vi "User_Change_Password.vi"(11 "User_Name":string caption="用  户  名") -> ()   [LabVIEW 2020]
panel:
  in  "Confirm Password":string caption="确认密码"
  in  "New Password":string caption="新  密  码"
  in  "Last Password":string caption="旧  密  码"
  in  "Ok":bool
  # "修改密码"
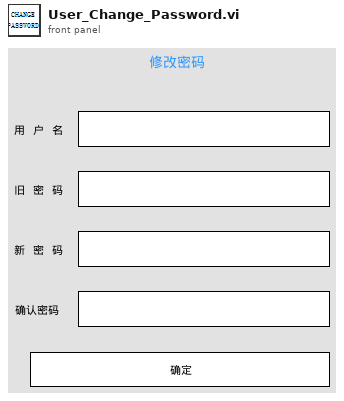
[diagram p1: front panel]
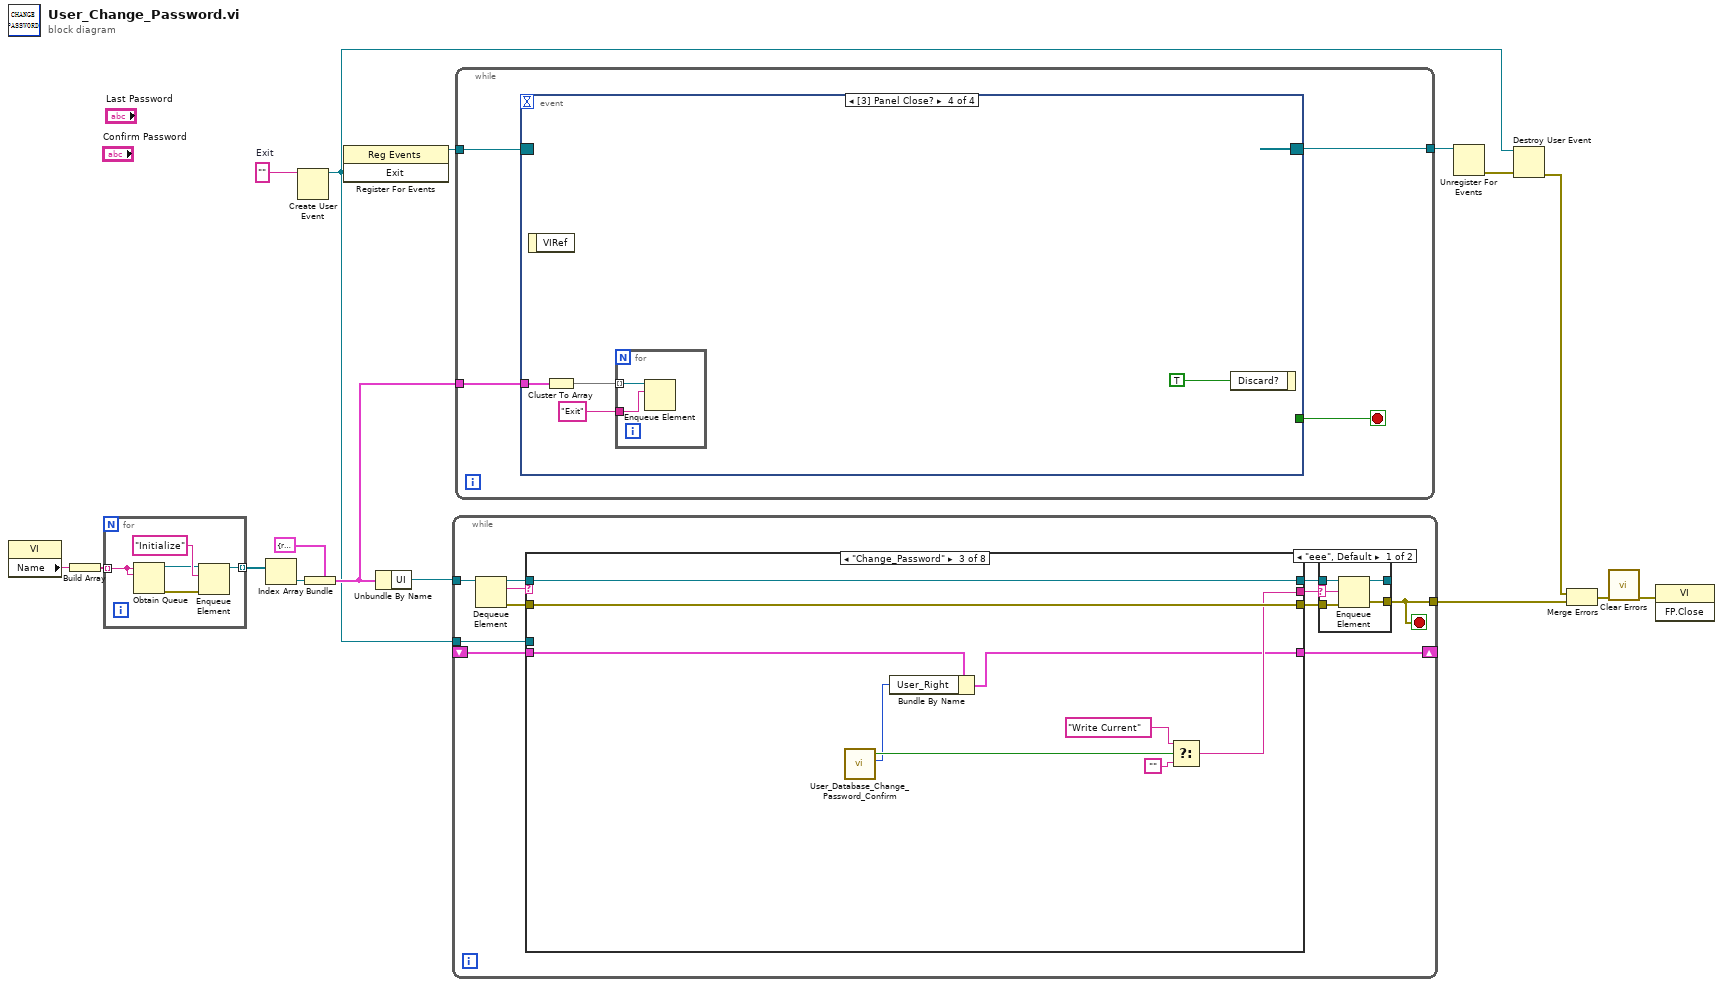
[diagram p0: block diagram]
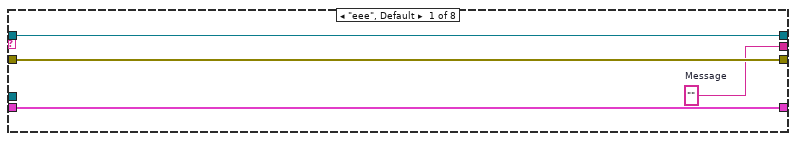
[diagram p3: hidden frame]
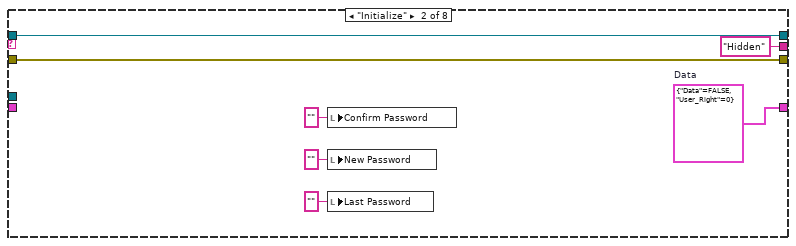
[diagram p4: hidden frame]
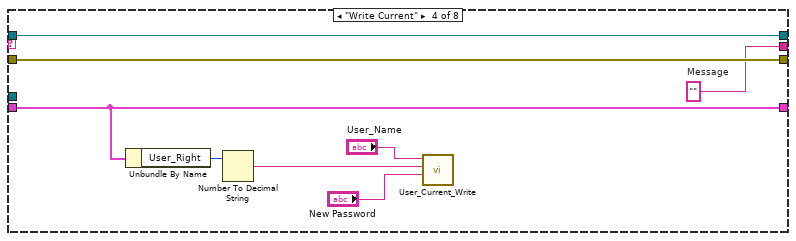
[diagram p5: hidden frame]
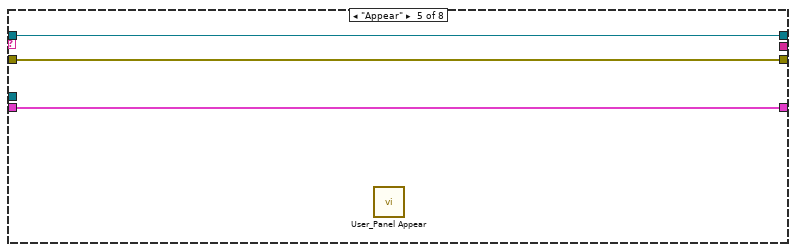
[diagram p6: hidden frame]
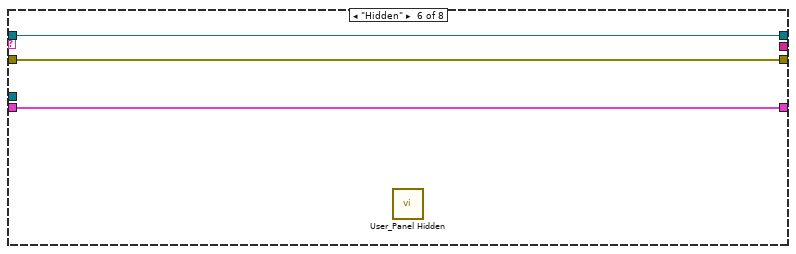
[diagram p7: hidden frame]
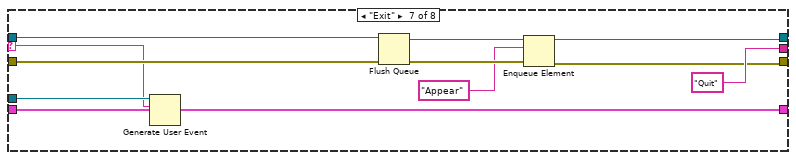
[diagram p8: hidden frame]
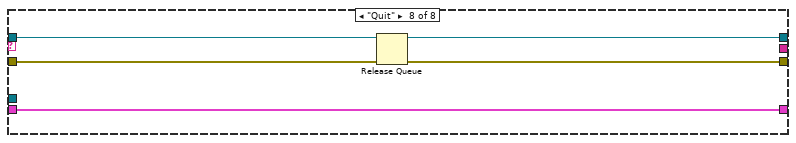
[diagram p9: hidden frame]
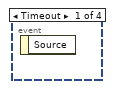
[diagram p10: hidden frame]
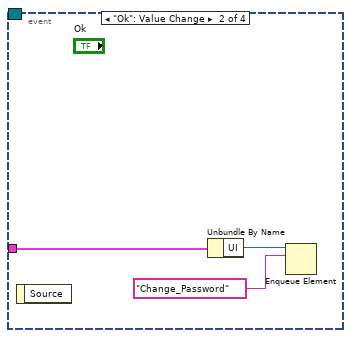
[diagram p11: hidden frame]
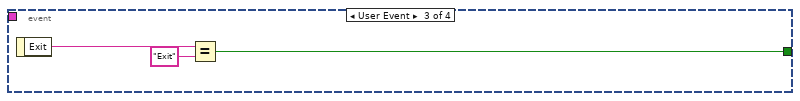
[diagram p12: hidden frame]
diagram:
  w2 = ""  # Exit
  n1 = property class="VI"() -> ("Name"=w12:string)  [unwired: 2 in, 2 out]
  n2 = Build Array(w12) -> (w13:string[])
  n3 = for {
    tunnel: w13 -> [w17] mode=indexing
    tunnel: [w18] -> w7 mode=indexing
    n4 = Obtain Queue(name (unnamed)=w17, element data type=w17) -> (queue out=w20:refnum<queue>, error out=w19:errorcluster)  [unwired: 3 in, 1 out]
    n5 = Enqueue Element(queue=w20, element="Initialize" ("元素"), error in (no error)=w19) -> (queue out=w18:refnum<queue>)  [unwired: 1 in, 2 out]
  }
  n6 = Index Array(array=w7) -> (element=w10:refnum<queue>)  [unwired: 1 in]
  n7 = Create User Event(user event datatype=w2) -> (user event=w6:refnum<user-event>)  [unwired: 1 in, 1 out]
  n8 = Bundle(cluster=cluster{"UI":refnum<queue>} {"UI"=refnum}, "UI"=w10) -> (w11:cluster{"UI":refnum<queue>})
  n9 = register-events(w6) -> (reference out=w3:refnum<event-registration>)  [unwired: 2 in, 1 out]
  n10 = Unbundle By Name(w11) -> ("UI"=w8:refnum<queue>)
  n11 = while {
    tunnel: w8 -> [w32]
    tunnel: [w22] -> w15
    shift-right: [w26] -> _
    shift-left: _ -> [w25]
    tunnel: w6 -> [w24]
    stop <- w22 stop-if-true
    n12 = Dequeue Element(queue=w32) -> (queue out=w31:refnum<queue>, element=w23:string, error out=w28:errorcluster)  [unwired: 2 in, 1 out]
    n13 = case shown="\"Change_Password\"" w23 {
      selector: w23 -> [_ _ _ _ _ _ w79 _]
      tunnel: w31 -> [w43 w50 w59 w67 w70 w73 w82 w88]
      tunnel: [w43 w50 w59 w67 w70 w73 w77 w88] -> w30
      tunnel: [w42 w49 w58 w66 w69 w72 w75 w85] -> w29
      tunnel: w28 -> [w42 w49 w58 w66 w69 w72 w81 w87]
      tunnel: [w41 "Hidden" ("Message") w54 w65 _ _ "Quit" ("Message") _] -> w27
      tunnel: [w40 w48 w51 w62 w68 w71 w84 w86] -> w26
      tunnel: w25 -> [w40 _ w53 w62 w68 w71 w84 w86]
      tunnel: w24 -> [_ _ _ _ _ _ w80 _]
      frame "eee", Default {
        w41 = ""  # Message
      }
      frame "Initialize" {
        w48 = cluster{"Data":bool, "User_Right":i32} {"Data"=FALSE, "User_Right"=0}  # Data
        n14 = local write "Confirm Password"("" ("Confirm Password")) -> ()
        n15 = local write "New Password"("" ("New Password")) -> ()
        n16 = local write "Last Password"("" ("Last Password")) -> ()
      }
      frame "Change_Password" {
        n17 = call "User_Database_Change_Password_Confirm.vi"() -> ("User_Right"=w52:i32, "OK"=w57:bool)  [unwired: 9 in, 1 out]
        n18 = Bundle By Name(cluster=w53, "User_Right"=w52) -> (w51:cluster{"Data":bool, "User_Right":i32})
        n19 = Select(t="Write Current" ("Message"), s=w57, f="") -> (s? t:f=w54:string)
      }
      frame "Write Current" {
        w65 = ""  # Message
        n20 = Unbundle By Name(w62) -> ("User_Right"=w61:i32)
        n21 = Number To Decimal String(number=w61) -> (decimal integer string=w60:string)  [unwired: 1 in]
        n22 = call "User_Current_Write.vi"("Password"="New Password", "User_Right"=w60, "Name"="User_Name") -> ()  [unwired: 8 in, 1 out]
      }
      frame "Appear" {
        n23 = call "User_Panel Appear.vi"() -> ()  [unwired: 11 in, 1 out]
      }
      frame "Hidden" {
        n24 = call "User_Panel Hidden.vi"() -> ()  [unwired: 11 in, 1 out]
      }
      frame "Exit" {
        n25 = Generate User Event(user event=w80, event data cluster=w79) -> ()  [unwired: 2 in, 2 out]
        n26 = Flush Queue(queue=w82, error in (no error)=w81) -> (queue out=w78:refnum<queue>, error out=w76:errorcluster)  [unwired: 1 out]
        n27 = Enqueue Element(queue=w78, element="Appear" ("元素"), error in (no error)=w76) -> (queue out=w77:refnum<queue>, error out=w75:errorcluster)  [unwired: 1 in, 1 out]
      }
      frame "Quit" {
        n28 = Release Queue(queue=w88, error in (no error)=w87) -> (error out=w85:errorcluster)  [unwired: 1 in, 2 out]
      }
    }
    n29 = case shown="\"eee\", Default" w27 {
      selector: w27 -> [w33 _]
      tunnel: w30 -> [w37 w39]
      tunnel: w29 -> [w36 w38]
      tunnel: [w35 w38] -> w22
      tunnel: [w34 w39] -> _
      frame "eee", Default {
        n30 = Enqueue Element(queue=w37, element=w33, error in (no error)=w36) -> (queue out=w34:refnum<queue>, error out=w35:errorcluster)  [unwired: 1 in, 1 out]
      }
      frame "" {
      }
    }
  }
  n31 = while {
    tunnel: w3 -> [w91]
    tunnel: [w90] -> w5
    tunnel: w11 -> [w89]
    stop <- w92 stop-if-true
    n32 = event shown="[3] Panel Close?" {
      selector: w91 -> [_ _ _ _]
      dyn-events: [_ _ _ _] -> w90
      timeout: _ -> [_ _ _ _]
      tunnel: [_ _ w97 _] -> w92
      tunnel: w89 -> [_ w93 _ w101]
      event Timeout {
        n33 = event-data() -> ()  [unwired: 1 in, 1 out]
      }
      event "Ok": Value Change {
        n34 = event-data() -> ()  [unwired: 1 in, 1 out]
        n35 = Unbundle By Name(w93) -> ("UI"=w95:refnum<queue>)
        n36 = Enqueue Element(queue=w95, element="Change_Password" ("元素")) -> ()  [unwired: 2 in, 3 out]
      }
      event User Event {
        n37 = event-data() -> ("Exit"=w98:string)  [unwired: 1 in]
        n38 = Equal?(x=w98, y="Exit") -> (x = y?=w97:bool)
      }
      event Panel Close? {
        n39 = event-data() -> ()  [unwired: 1 in, 1 out]
        n40 = Cluster To Array(cluster=w101) -> (array=w100:refnum<queue>[])
        n41 = for {
          tunnel: w100 -> [w104] mode=indexing
          tunnel: "Exit" ("元素") -> [w103]
          n42 = Enqueue Element(queue=w104, element=w103) -> ()  [unwired: 2 in, 3 out]
        }
        n43 = event-data("Discard?"=TRUE ("放弃？")) -> ()  [unwired: 1 in, 1 out]
      }
    }
  }
  n44 = Unregister For Events(event registration refnum=w5) -> (error out=w4:errorcluster)  [unwired: 1 in]
  n45 = Destroy User Event(user event=w6, error in=w4) -> (error out=w14:errorcluster)
  n46 = Merge Errors(w14, w15) -> (w16:errorcluster)
  n47 = call <vilib>:"Clear Errors.vi"("error in (no error)"=w16) -> ("error out"=w1:errorcluster)  [unwired: 5 in, 1 out]
  n48 = invoke class="VI" method="FP.Close"(error in=w1) -> ()  [unwired: 2 in, 3 out]
